vi "Read Back Vibration_Micriphone_Encoder Signal.vi"() -> ()   [LabVIEW 2021]
uses:
  <vilib>/express/express analysis/Spectral/Block/exnSpectralBlock spectral measurements power poly.vi
  <vilib>/express/express analysis/Spectral/Block/exnSpectralBlock spectral measurements power DDT.vi
  <vilib>/express/express analysis/Spectral/XNode/ExpressSpectralMeasurementsBlockNode.xnode
panel:
  out "Time per Loop":dbl
  in  "Samps":dbl=100.0 caption="Numbers of Sample"
  in  "Sample Rate":dbl=1000.0
  in  "File Path":path
  in  "Save Button":bool
  out "Spec Total":dynamicdata(graph)
  in  "Upper Cut-Off 3":dbl=400.0 caption="Upper Cut-Off"
  in  "Lower Cut-Off 3":dbl=100.0 caption="Lower Cut-Off"
  out "Microphone":dynamicdata(graph)
  in  "Upper Cut-Off 2":dbl=400.0 caption="Upper Cut-Off"
  in  "Lower Cut-Off 2":dbl=100.0 caption="Lower Cut-Off"
  out "Vibration Y":dynamicdata(graph)
  out "Vibration X":dynamicdata(graph)
  out "ai2 Overall":waveform(dbl)(graph)
  out "ai1 Overall":waveform(dbl)(graph)
  out "ai0 Overall":waveform(dbl)(graph)
  in  "Time":dbl(slide) step=0.1 scale=-1.0..11.100000000000001
  in  "Lower Cut-Off":dbl=100.0
  in  "Upper Cut-Off":dbl=400.0
  in  "stop":bool
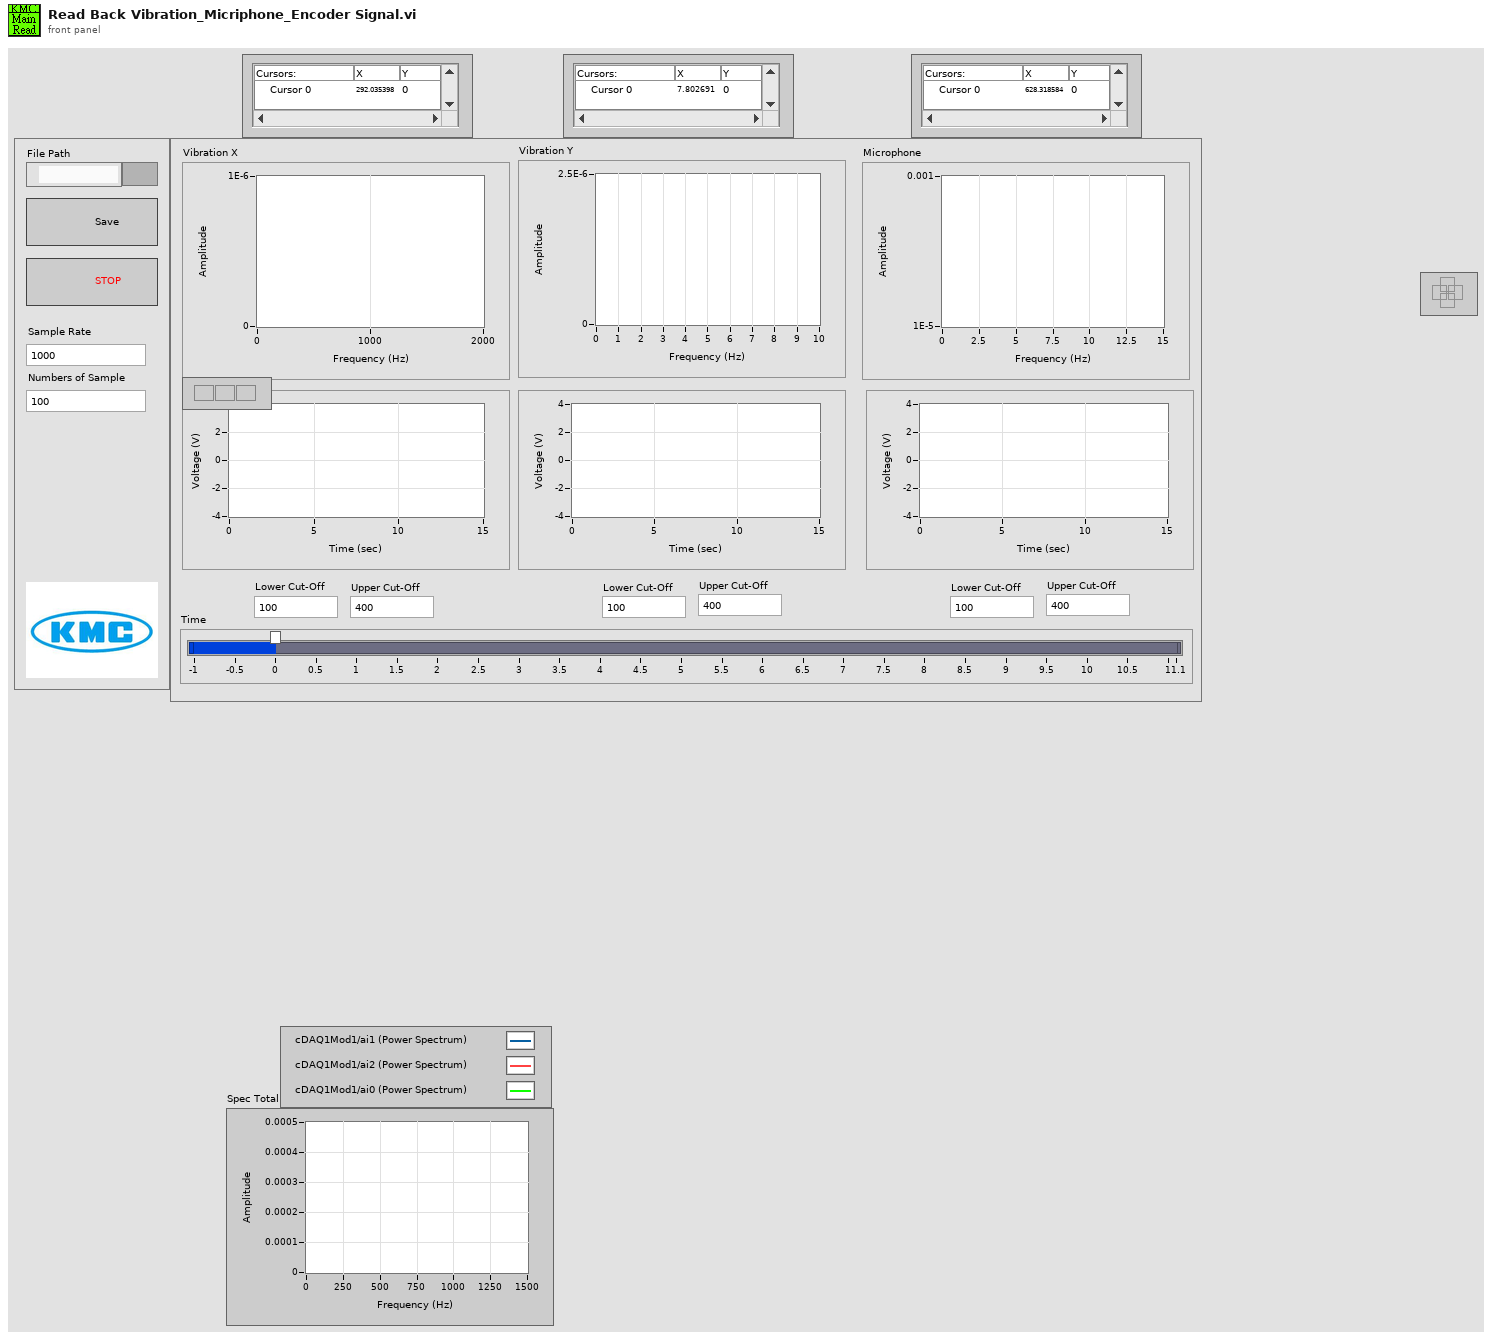
[diagram p1: front panel]
types:
  T1 = enum16{"open", "replace", "create", "open or create", "replace or create", "replace or create with confirmation"}
  T2 = cluster{"averaging mode":u16, "weighting mode":u16, "number of averages":u32}
  T3 = cluster{"dB On (F)":bool, "unwrap phase (F)":bool, "convert to degree (F)":bool}
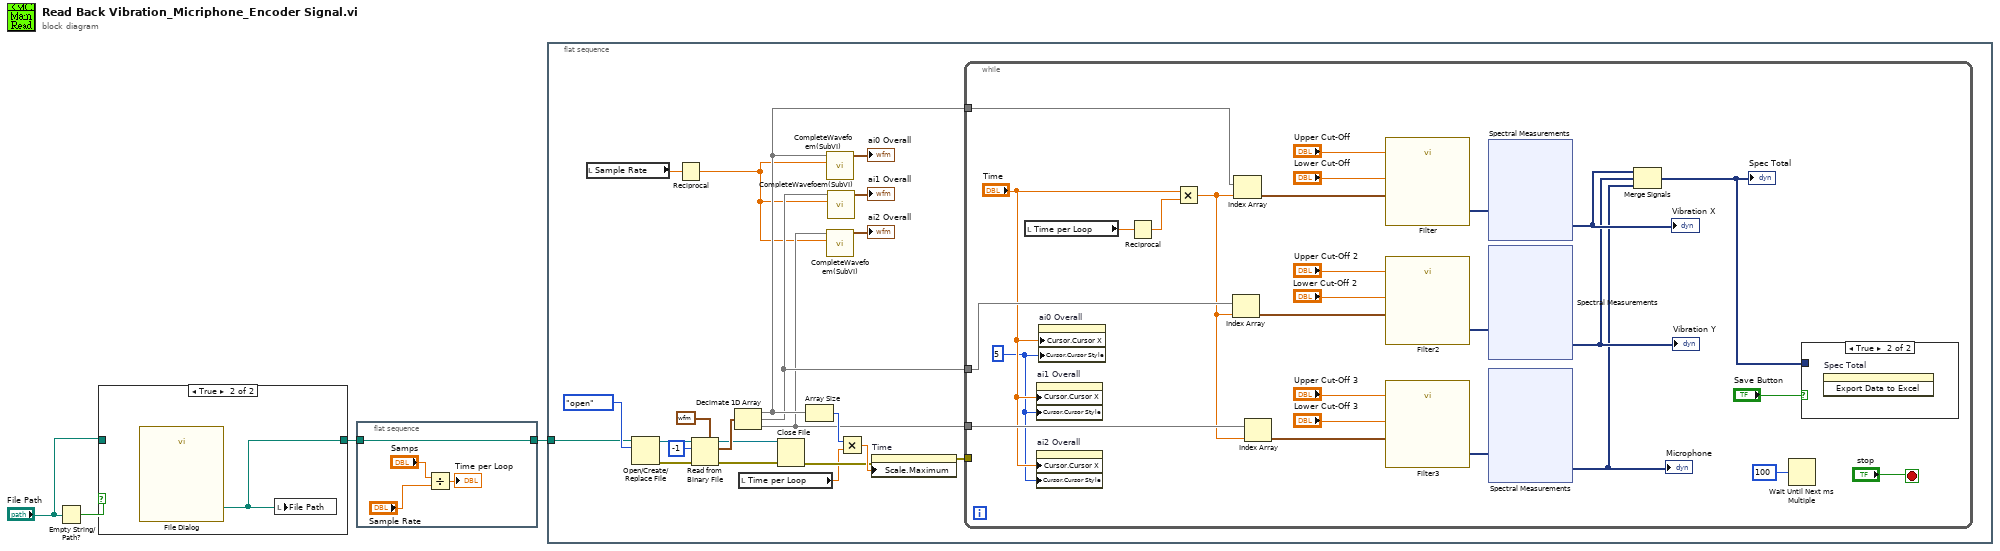
[diagram p0: block diagram]
diagram:
  n1 = Empty String/Path?(string/path="File Path") -> (empty?=w4:bool)
  n2 = case shown="True" w4 {
    tunnel: "File Path" -> [w5 _]
    tunnel: [w5 w6] -> w1
    frame False {
    }
    frame True {
      n3 = call "File Dialog"() -> ("selected path"=w6:path)  [unwired: 12 in, 3 out]
      n4 = local write "File Path"(w6) -> ()
    }
  }
  n5 = flat-sequence {
    tunnel: [w7] -> w2
    tunnel: w1 -> [w7]
    frame #0 {
      n6 = Divide(x="Samps", y="Sample Rate") -> (x/y=→"Time per Loop":dbl)
    }
  }
  n7 = flat-sequence {
    tunnel: w2 -> [w13]
    frame #0 {
      n8 = local read "Sample Rate"() -> (w12:dbl)
      n9 = Open/Create/Replace File(file path (use dialog)=w13, operation (0:open)=T1."open") -> (refnum out=w26:refnum<file>, error out=w25:errorcluster)  [unwired: 4 in, 1 out]
      n10 = Reciprocal(x=w12) -> (1/x=w11:dbl)
      n11 = Read from Binary File(5:waveform(dbl) {"t0"=timestamp(0 s since 1904-01-01), "dt"=1.0, "Y"=[]} ("transposed array"), 8:w25, 10:-1 ("count (1)"), 11:w26) -> (0:w23:errorcluster, 2:w29:waveform(dbl)[], 3:w24:refnum<file>)  [unwired: 2 in, 1 out]
      n12 = Decimate 1D Array(w29) -> (w21:waveform(dbl)[], w19:waveform(dbl)[], w17:waveform(dbl)[])
      n13 = local read "Time per Loop"() -> (w14:dbl)
      n14 = Close File(refnum=w24, error in=w23) -> (error out=w22:errorcluster)  [unwired: 1 out]
      n15 = Array Size(array=w21) -> (size(s)=w30:i32)
      n16 = call "CompleteWavefoem(SubVI).vi"("dt"=w11, "Array"=w21) -> ("Waveform"=→"ai0 Overall":waveform(dbl))  [unwired: 9 in]
      n17 = call "CompleteWavefoem(SubVI).vi"("dt"=w11, "Array"=w17) -> ("Waveform"=→"ai2 Overall":waveform(dbl))  [unwired: 9 in]
      n18 = call "CompleteWavefoem(SubVI).vi"("dt"=w11, "Array"=w19) -> ("Waveform"=→"ai1 Overall":waveform(dbl))  [unwired: 9 in]
      n19 = Multiply(x=w30, y=w14) -> (x*y=w31:dbl)
      n20 = property on="Time" class="Slide (strict)"(error in=w22, "Scale.Maximum"=w31) -> (error out=w15:errorcluster)  [unwired: 1 in, 1 out]
      n21 = while {
        tunnel: w21 -> [w55]
        tunnel: w19 -> [w48]
        tunnel: w17 -> [w44]
        tunnel: w15 -> [_]
        stop <- "stop" stop-if-true
        w41 = u8 5 ("Cursor.Cursor Style")
        n22 = local read "Time per Loop"() -> (w34:dbl)
        n23 = property on="ai1 Overall" class="WFGraph (strict)"("Cursor.Cursor X"="Time", "Cursor.Cursor Style"=w41) -> ()  [unwired: 2 in, 2 out]
        n24 = property on="ai2 Overall" class="WFGraph (strict)"("Cursor.Cursor X"="Time", "Cursor.Cursor Style"=w41) -> ()  [unwired: 2 in, 2 out]
        n25 = property on="ai0 Overall" class="WFGraph (strict)"("Cursor.Cursor X"="Time", "Cursor.Cursor Style"=w41) -> ()  [unwired: 2 in, 2 out]
        n26 = Reciprocal(x=w34) -> (1/x=w33:dbl)
        n27 = Multiply(x="Time", y=w33) -> (x*y=w43:dbl)
        n28 = Index Array(array=w48, index=w43) -> (element=w51:waveform(dbl))
        n29 = Index Array(array=w55, index=w43) -> (element=w54:waveform(dbl))
        n30 = Index Array(array=w44, index=w43) -> (element=w45:waveform(dbl))
        n31 = call "Filter"("Lower Cut-Off"="Lower Cut-Off", "Upper Cut-Off"="Upper Cut-Off", "Signal"=w54) -> ("Filtered Signal"=w53:dynamicdata)  [unwired: 7 in, 1 out]
        n32 = call "Filter2"("Lower Cut-Off"="Lower Cut-Off 2", "Upper Cut-Off"="Upper Cut-Off 2", "Signal"=w51) -> ("Filtered Signal"=w52:dynamicdata)  [unwired: 7 in, 1 out]
        n33 = call "Filter3"("Lower Cut-Off"="Lower Cut-Off 3", "Upper Cut-Off"="Upper Cut-Off 3", "Signal"=w45) -> ("Filtered Signal"=w40:dynamicdata)  [unwired: 7 in, 1 out]
        n34 = xnode "Spectral Measurements"("Signals"=w53) -> ("Power Spectrum"=w39:dynamicdata)  [unwired: 1 in, 1 out]
        "Vibration X" <- w39
        n35 = xnode "Spectral Measurements"("Signals"=w52) -> ("Power Spectrum"=w38:dynamicdata)  [unwired: 1 in, 1 out]
        "Vibration Y" <- w38
        n36 = xnode "Spectral Measurements"("Signals"=w40) -> ("Power Spectrum"=w37:dynamicdata)  [unwired: 1 in, 1 out]
        "Microphone" <- w37
        n37 = Merge Signals(w39, w38, w37) -> (w35:dynamicdata)
        "Spec Total" <- w35
        n38 = Wait Until Next ms Multiple(millisecond multiple=u32 100 ("milliseconds to wait")) -> ()  [unwired: 1 out]
        n39 = case shown="True" "Save Button" {
          tunnel: w35 -> [_ _]
          frame False {
          }
          frame True {
            n40 = invoke on="Spec Total" class="WFGraph (strict)" method="Export Data to Excel"() -> ()  [unwired: 3 in, 3 out]
          }
        }
      }
    }
  }
